vi "Write Ethernet Config.vi"() -> (0 "error out":errorcluster)   [LabVIEW 2020]
panel:
  in  "Values (other)":dbl[](array[numeric])=[1.0] format="%.2f"
  in  "Names (other)":string[](array[string])=["ETHERNET_DHCP_ENABLE_DEFAULT"]
  in  "IP String Values":string[](array[string])=["192.168.1.207", "255.255.255.0", "192.168.1.1"]
  out "Error String":string
  out "ConnectionType Out":i32
  out "DeviceType Out":i32
  in  "Identifier":string="LJM_idANY"
  in  "ConnectionType":string="LJM_ctANY"
  in  "DeviceType":string="LJM_dtANY"
  out "Values (IP)":dbl[](array[numeric]) format="%.2f"
  in  "Names (IP)":string[](array[string])=["ETHERNET_IP_DEFAULT", "ETHERNET_SUBNET_DEFAULT", "ETHERNET_GATEWAY_DEFAULT"]
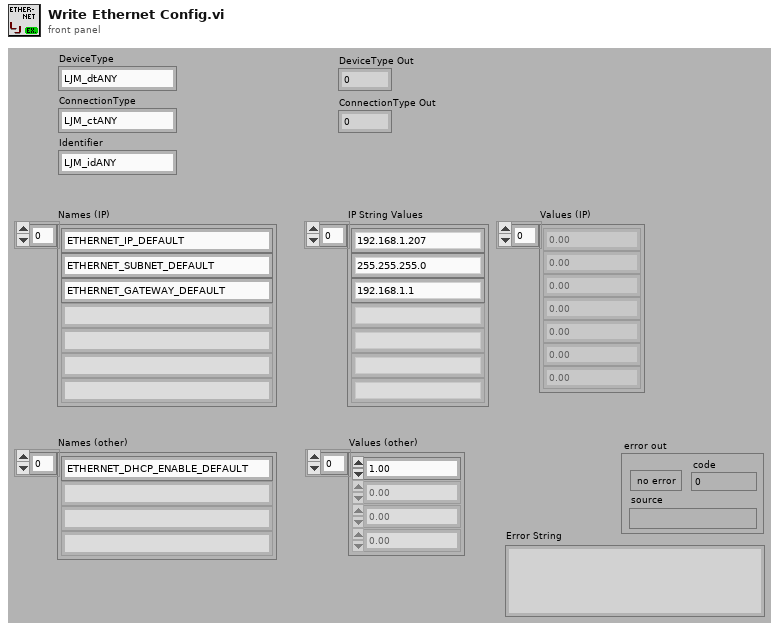
[diagram p1: front panel]
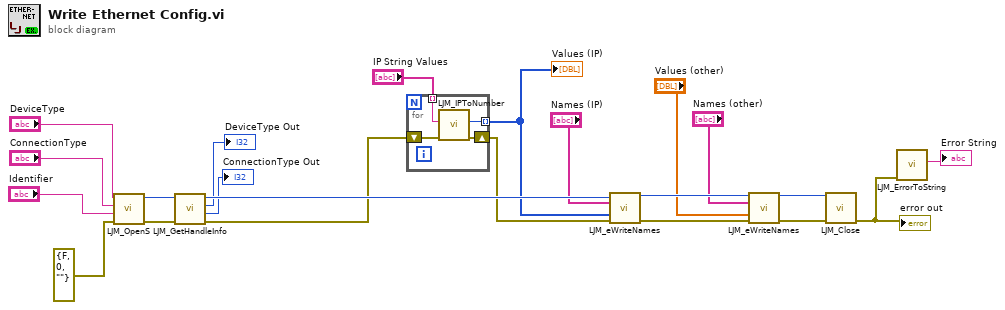
[diagram p0: block diagram]
diagram:
  n1 = call "LJM_OpenS.vi"("error in"=errorcluster {"status"=FALSE, "code"=0, "source"=""} ("error in (no error)"), "Identifier"="Identifier", "ConnectionType"="ConnectionType", "DeviceType"="DeviceType") -> ("error out"=w21:errorcluster, "Handle"=w20:i32)  [unwired: 6 in]
  n2 = call "LJM_GetHandleInfo.vi"("error in"=w21, "Handle In"=w20) -> ("error out"=w5:errorcluster, "ConnectionType"=→"ConnectionType Out":i32, "DeviceType"=→"DeviceType Out":i32, "Handle Out"=w19:i32)  [unwired: 2 in, 4 out]
  n3 = for {
    shift-right: [w25] -> w4
    shift-left: w5 -> [w26]
    tunnel: "IP String Values" -> [w24] mode=indexing
    tunnel: [w23] -> w2 mode=indexing
    n4 = call "LJM_IPToNumber.vi"("error in"=w26, "IPv4String"=w24) -> ("error out"=w25:errorcluster, "Number"=w23:u32)  [unwired: 8 in]
  }
  "Values (IP)" <- w2
  n5 = call "LJM_eWriteNames.vi"("Handle In"=w19, "aNames"="Names (IP)", "aValuesIn"=w2, "error in"=w4) -> ("Handle Out"=w10:i32, "error out"=w9:errorcluster)  [unwired: 9 in, 1 out]
  n6 = call "LJM_eWriteNames.vi"("Handle In"=w10, "aNames"="Names (other)", "aValuesIn"="Values (other)", "error in"=w9) -> ("Handle Out"=w7:i32, "error out"=w6:errorcluster)  [unwired: 9 in, 1 out]
  n7 = call "LJM_Close.vi"("error in"=w6, "Handle"=w7) -> ("error out"=w13:errorcluster)  [unwired: 9 in]
  "error out" <- w13
  n8 = call "LJM_ErrorToString.vi"("error in"=w13) -> ("String"=→"Error String":string)  [unwired: 10 in]
